vi "Set NI_XNET_CAN_Bus_Monitor_API SetStreamingFilter Response.vi"(7 "Streaming? (F)":bool, 8 "error in (no error)":errorcluster, 10 "Message Data":T1, 11 "gRPCid in":T3) -> (0 "error out":errorcluster)   [LabVIEW 2025, in "xnet_can_bus_monitor_api_server.lvlib" / "NI_XNET_CAN_Bus_Monitor_API.lvclass"]
uses:
  NI_XNET_CAN_Bus_Monitor_API.lvclass
  <vilib>/gRPC/LabVIEW gRPC Library/Shared/grpcId.ctl
  NI_XNET_CAN_Bus_Monitor_API.lvclass/NI_XNET_CAN_Bus_Monitor_API.ctl
  xnet_can_bus_monitor_api_server.lvlib
  <vilib>/gRPC/LabVIEW gRPC Library/grpc-lvsupport-release.lvlib
  RPC Messages/ni_xnet_can_bm_api_ErrorInfo.ctl
  RPC Messages/ni_xnet_can_bm_api_SetStreamingFilterReply.ctl
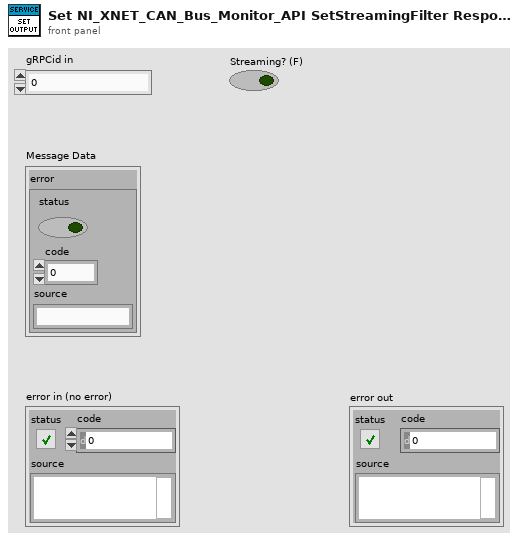
[diagram p1: front panel]
types:
  T1 = typedef "xnet_can_bus_monitor_api_server.lvlib/ni_xnet_can_bm_api_SetStreamingFilterReply.ctl" = cluster{"error":T2}
  T2 = typedef "xnet_can_bus_monitor_api_server.lvlib/ni_xnet_can_bm_api_ErrorInfo.ctl" = errorcluster
  T3 = typedef "grpc-lvsupport-release.lvlib/grpcId.ctl" = u64
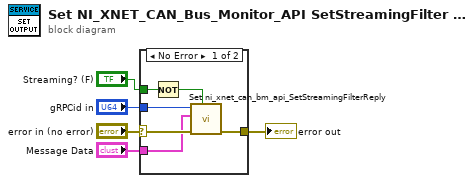
[diagram p0: block diagram]
diagram:
  n1 = case shown="No Error" "error in (no error)" {
    selector: "error in (no error)" -> [w11 w12]
    tunnel: [w9 w12] -> w4
    tunnel: "gRPCid in" -> [w10 _]
    tunnel: "Message Data" -> [w8 _]
    tunnel: "Streaming? (F)" -> [w7 _]
    frame No Error {
      n2 = Not(x=w7) -> (.not. x?=w6:bool)
      n3 = call "Set ni_xnet_can_bm_api_SetStreamingFilterReply.vi"("Complete Call (T)"=w6, "error in (no error)"=w11, "package_templatemessage"=w8, "gRPCid"=w10) -> ("error out"=w9:errorcluster)  [unwired: 7 in]
    }
    frame Error {
    }
  }
  "error out" <- w4
